vi "SwapInstanceVIUnusedName2 66.vi"(6 "Bindata & descr in":T1, 7 "type":u32, 8 "error in (no error)":errorcluster, 9 "dims":u8=3 min=1 max=3, 11 "kwarg_name":string="testarg") -> (0 "error out":errorcluster, 1 "Array 3D":u32[][][](array[numeric]), 2 "Array 2D":u32[][](array[numeric]), 3 "Array 1D":u32[](array[numeric]), 4 "Bindata & descr out":T1, 5 "bindata":u8[](array[numeric]))   [LabVIEW 2018]
uses:
  Bindata&description.ctl
  Bindata description.ctl
  78faac7b-e721-4ead-a4fd-ab2be5276b46.vi
  63a393ed-cd6b-4293-bc0b-fa0c8608a16b.vi
  f41a4835-c689-4cbf-8256-ee0d504a709d.vi
  99de1ede-1565-4a86-9063-3b96e501d90c.vi
  63a393ed-cd6b-4293-bc0b-fa0c8608a16b.vi/74036071-1ecc-4cd4-8bec-9b35d7948a7d.vi
  f41a4835-c689-4cbf-8256-ee0d504a709d.vi/8af0878c-0fd6-425c-b85b-5e433a2e138b.vi
  99de1ede-1565-4a86-9063-3b96e501d90c.vi/fee80d8b-489a-4844-a9b8-9fba77535efb.vi
  63a393ed-cd6b-4293-bc0b-fa0c8608a16b.vi/74036071-1ecc-4cd4-8bec-9b35d7948a7d.vi/222ed911-f5aa-4580-bdaf-ef98fed1d6eb.vi
  f41a4835-c689-4cbf-8256-ee0d504a709d.vi/8af0878c-0fd6-425c-b85b-5e433a2e138b.vi/4227abe2-efde-4c22-8247-c9382135964d.vi
  99de1ede-1565-4a86-9063-3b96e501d90c.vi/fee80d8b-489a-4844-a9b8-9fba77535efb.vi/13ed2b74-6544-4f29-b0d5-37a7d7e9441c.vi
  63a393ed-cd6b-4293-bc0b-fa0c8608a16b.vi/74036071-1ecc-4cd4-8bec-9b35d7948a7d.vi/222ed911-f5aa-4580-bdaf-ef98fed1d6eb.vi/0396df40-b741-41fe-9323-018ec49dbcf7.vi
  f41a4835-c689-4cbf-8256-ee0d504a709d.vi/8af0878c-0fd6-425c-b85b-5e433a2e138b.vi/4227abe2-efde-4c22-8247-c9382135964d.vi/50413334-d671-4bc3-a1ba-467fee9f2375.vi
  99de1ede-1565-4a86-9063-3b96e501d90c.vi/fee80d8b-489a-4844-a9b8-9fba77535efb.vi/13ed2b74-6544-4f29-b0d5-37a7d7e9441c.vi/4b0ca402-d759-4749-bb03-bb3ae84f631f.vi
  check ID validity.vi
  LV-Julia_ZMQ-Roundtrip_lib.lvlib
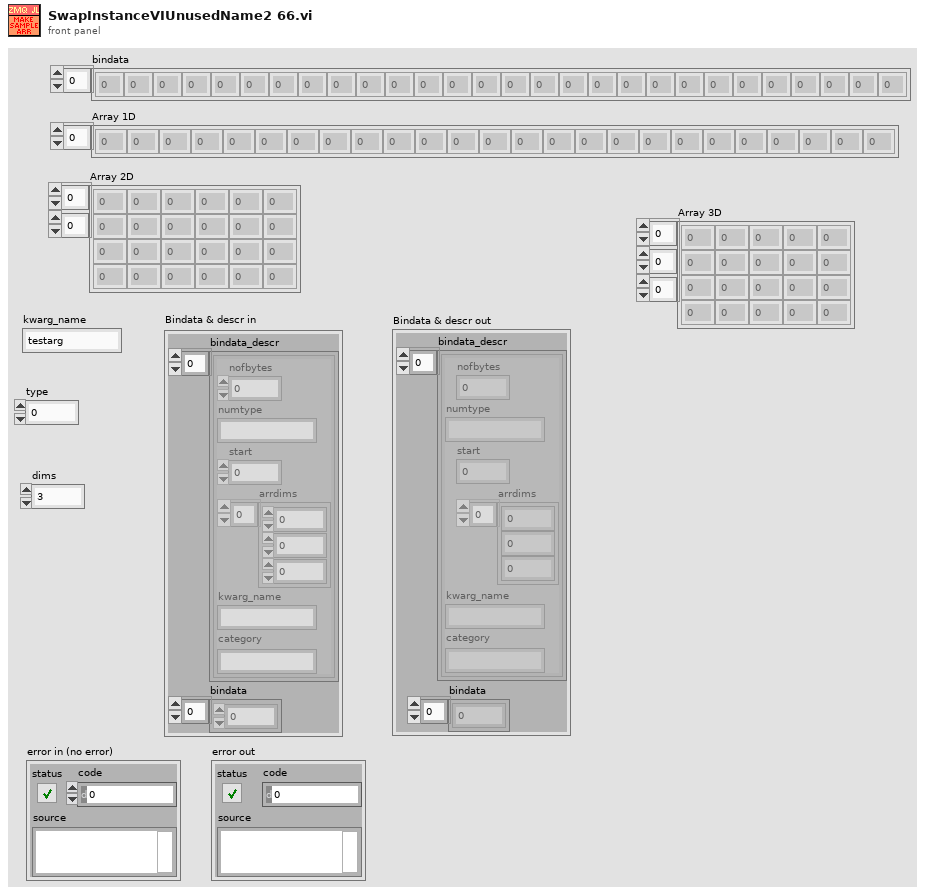
[diagram p1: front panel]
types:
  T1 = typedef "Bindata&description.ctl" = cluster{"bindata_descr":T2[], "bindata":u8[]}
  T2 = typedef "LV-Julia_ZMQ-Roundtrip_lib.lvlib/Bindata description.ctl" = cluster{"nofbytes":i32, "numtype":string, "start":i32, "arrdims":i32[], "kwarg_name":string, "category":string}
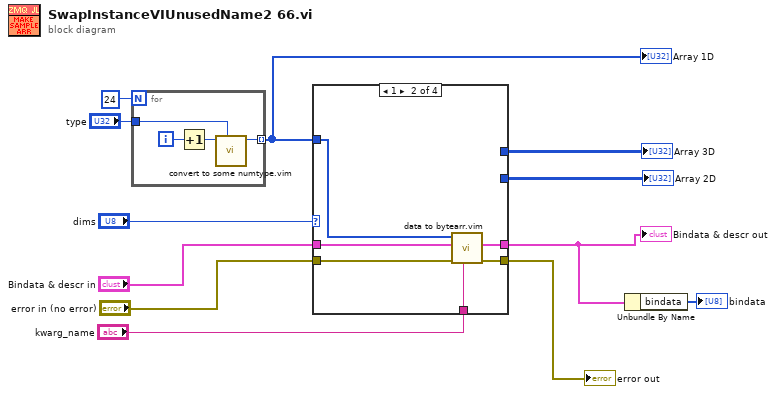
[diagram p0: block diagram]
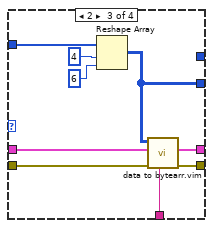
[diagram p3: hidden frame]
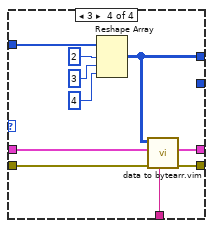
[diagram p4: hidden frame]
diagram:
  n1 = for {
    N: 24 -> [_]
    tunnel: [w14] -> w11 mode=indexing
    tunnel: "type" -> [w13]
    i -> [w16]
    n2 = Increment(x=w16) -> (x+1=w15:i32)
    n3 = call "convert to some numtype.vim"("type"=w13, "Numeric in"=w15) -> ("Numeric out"=w14:u32)  [unwired: 9 in]
  }
  "Array 1D" <- w11
  n4 = case shown="1" "dims" {
    tunnel: [_ _ _ w42] -> w12
    tunnel: w11 -> [_ w23 w30 w38]
    tunnel: "kwarg_name" -> [_ w22 w29 w37]
    tunnel: "error in (no error)" -> [w17 w21 w28 w36]
    tunnel: [w17 w20 w27 w35] -> w5
    tunnel: [_ w19 w26 w34] -> w2
    tunnel: [_ _ w25 _] -> w4
    tunnel: "Bindata & descr in" -> [_ w18 w24 w33]
    frame 0, Default {
    }
    frame 1 {
      n5 = call "data to bytearr.vim"("kwarg_name"=w22, "error in (no error)"=w21, "Bindata & descr in"=w18, "data in"=w23) -> ("error out"=w20:errorcluster, "Bindata & descr out"=w19:T1)  [unwired: 5 in, 1 out]
    }
    frame 2 {
      n6 = Reshape Array(w30, 4 ("dimension size"), 6 ("dimension size")) -> (w25:u32[][])
      n7 = call "data to bytearr.vim"("kwarg_name"=w29, "error in (no error)"=w28, "Bindata & descr in"=w24, "data in"=w25) -> ("error out"=w27:errorcluster, "Bindata & descr out"=w26:T1)  [unwired: 5 in, 1 out]
    }
    frame 3 {
      n8 = Reshape Array(w38, 2 ("dimension size"), 3 ("dimension size"), 4 ("dimension size")) -> (w42:u32[][][])
      n9 = call "data to bytearr.vim"("kwarg_name"=w37, "error in (no error)"=w36, "Bindata & descr in"=w33, "data in"=w42) -> ("error out"=w35:errorcluster, "Bindata & descr out"=w34:T1)  [unwired: 5 in, 1 out]
    }
  }
  "Array 3D" <- w12
  "Bindata & descr out" <- w2
  "error out" <- w5
  "Array 2D" <- w4
  n10 = Unbundle By Name(w2) -> ("bindata"=→"bindata":u8[])
